vi "Exercises_4-2.vi"() -> ()   [LabVIEW 2014]
panel:
  out "Number of iteration":i32
  out "Current Number":dbl format="%#.0f"
  in  "Number to Match":dbl=50.0 min=0.0 max=1000.0 step=1.0 format="%#.0g"
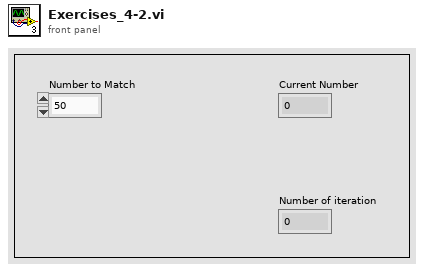
[diagram p1: front panel]
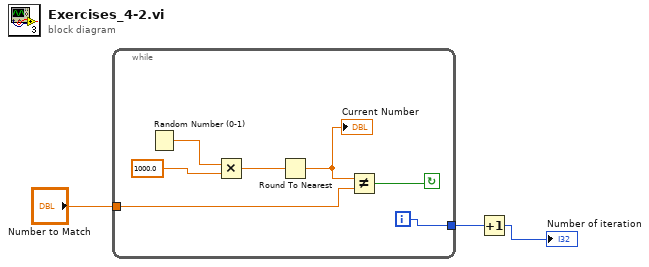
[diagram p0: block diagram]
diagram:
  n1 = while {
    tunnel: "Number to Match" -> [w7]
    tunnel: [w4] -> w2
    i -> [w4]
    stop <- w6 continue-if-true
    n2 = Random Number (0-1)() -> (number: 0 to 1=w9:dbl)
    n3 = Multiply(x=w9, y=1000.0) -> (x*y=w8:dbl)
    n4 = Round To Nearest(number=w8) -> (nearest integer value=w5:dbl)
    "Current Number" <- w5
    n5 = Not Equal?(x=w5, y=w7) -> (x != y?=w6:bool)
  }
  n6 = Increment(x=w2) -> (x+1=→"Number of iteration":i32)
